vi "ConfigClock.vi"(8 "error in (no error)":errorcluster, 11 "DAQmx_Single in":refnum<class "DaqMx_Single.lvclass">) -> (0 "error out":errorcluster, 3 "DAQmx_Single out":refnum<class "DaqMx_Single.lvclass">)   [LabVIEW 2014, in "FgenPlugins.lvlib" / "DaqMx_Single.lvclass"]
uses:
  DaqMx_Single.lvclass
  NiPxi6733Class/NiPxi6733.lvclass/NiPxi6733.ctl
  FgenPluginBaseClass/FgenPluginsBase.lvclass/FgenPluginsBase.ctl
  NiPxi6733Class/Accessors/Read Timebase.vi
  NiPxi6733Class/Accessors/Read SampleRate.vi
  FgenPluginBaseClass/Accessors/Read Channels.vi
  <resource>/objmgr/daqmx.rc
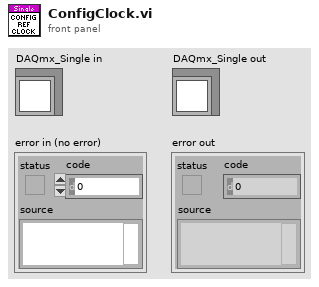
[diagram p1: front panel]
types:
  T1 = typedef "FgenPlugins.lvlib/NiPxi6733.lvclass/Timebase.ctl" = cluster{"source":string, "rate":dbl}
  T2 = typedef "FgenPlugins.lvlib/Channel.ctl" = cluster{"Name":string, "Enabled":bool, "Operation":enum16{"Continuous", "Burst"}, "Impedance (50)":dbl, "Handle":string, "Connected":bool, "Mode (Function)":enum16{"Function", "Arbitrary", "Sequence"}}
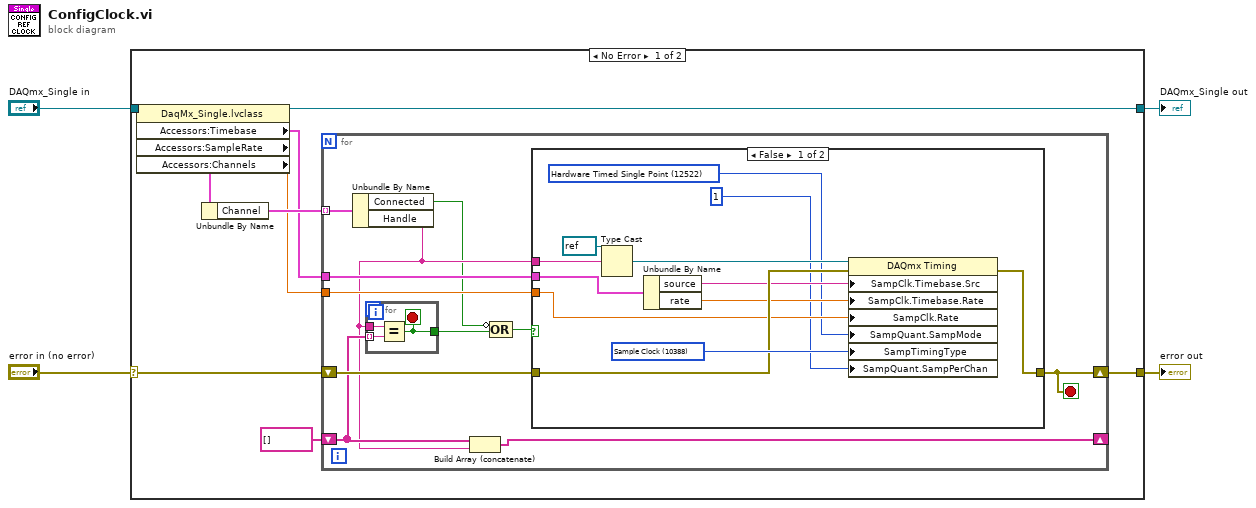
[diagram p0: block diagram]
diagram:
  n1 = case shown="No Error" "error in (no error)" {
    selector: "error in (no error)" -> [w12 w42]
    tunnel: [w9 w42] -> w3
    tunnel: [w5 w41] -> w1
    tunnel: "DAQmx_Single in" -> [w13 w41]
    frame No Error {
      n2 = property class="DaqMx_Single.lvclass"(reference=w13) -> (reference out=w5:refnum<class "DaqMx_Single.lvclass">, "Accessors:Timebase"=w6:T1, "Accessors:SampleRate"=w7:dbl, "Accessors:Channels"=w8:cluster{"Count":u16, "Channel":T2[]})  [unwired: 1 in, 1 out]
      n3 = Unbundle By Name(w8) -> ("Channel"=w11:T2[])
      n4 = for {
        shift-right: [w22] -> w9
        shift-left: w12 -> [w24]
        tunnel: w11 -> [w19] mode=indexing
        tunnel: w7 -> [w23]
        shift-right: [w20] -> _
        shift-left: string[] [] -> [w21]
        tunnel: w6 -> [w18]
        stop <- w22 stop-if-true
        n5 = Unbundle By Name(w19) -> ("Connected"=w15:bool, "Handle"=w17:string)
        n6 = for {
          tunnel: w21 -> [w40] mode=indexing
          tunnel: w17 -> [w39]
          tunnel: [w38] -> w16
          stop <- w38 stop-if-true
          n7 = Equal?(x=w39, y=w40) -> (x = y?=w38:bool)
        }
        n8 = Build Array (concatenate)(w21, w17) -> (w20:string[])
        n9 = Compound Arithmetic op=OR(invert w15, w16) -> (w14:bool)
        n10 = case shown="False" w14 {
          tunnel: w24 -> [w31 w37]
          tunnel: w17 -> [w35 _]
          tunnel: w23 -> [w28 _]
          tunnel: [w30 w37] -> w22
          tunnel: w18 -> [w32 _]
          frame False {
            w26 = 12522 items=["Finite Samples"=10178, "Continuous Samples"=10123, "Hardware Timed Single Point"=12522] ("sample mode")
            w33 = 10388 items=["Sample Clock"=10388, "Burst Handshake"=12548, "Handshake"=10389, "Implicit"=10451, "On Demand"=10390, "Change Detection"=12504, "Pipelined Sample Clock"=14668] ("SampTimingType")
            n11 = Type Cast(type=refnum<k21> refnum ("DAQmx Task Name"), x=w35) -> (*(type *) &x=w34:refnum<k21>)
            n12 = Unbundle By Name(w32) -> ("source"=w27:string, "rate"=w29:dbl)
            n13 = property class="DAQmx Timing"(reference=w34, error in=w31, "SampClk.Timebase.Src"=w27, "SampClk.Timebase.Rate"=w29, "SampClk.Rate"=w28, "SampQuant.SampMode"=w26, "SampTimingType"=w33, "SampQuant.SampPerChan"=1 ("samples per channel")) -> (error out=w30:errorcluster)  [unwired: 1 out]
          }
          frame True {
          }
        }
      }
    }
    frame Error {
    }
  }
  "error out" <- w3
  "DAQmx_Single out" <- w1
